vi "MCP4725 Generate and Read Example 4.vi"(8 "Error In":errorcluster) -> (0 "Error Out":errorcluster)   [LabVIEW 2014]
doc: "This example produces stepped triangle wave on output in loop, there's no timing inside while loop so it's running as fast as it can, at test computer signal has frequency 440Hz and consists from 12 samples, so we are able to produce this fast signals at most."
uses:
  LabVIEW-Universal-Transcriptor-MCP4725/MCP4725.lvclass
  <vilib>/LabVIEW Universal Transcriptor/LabVIEW to Arduino Transcriptor/Transcriptors/System API/Serial println string.vi
panel:
  # "This example produces stepped triangle wave on output in loop, there's no timing inside while loop so it's running as fast as it can, at test computer signal has frequency 440Hz and consists from 12 samples, so we are able to produce this fast signals at most.\n\nWiring:\n  Arduino Nano  |  MCP4725 module\n  -----------------------------------------\n          VCC        |           +5V\n          GND        |           GND\n          A4           |           SDA\n          A5           |           SCL"
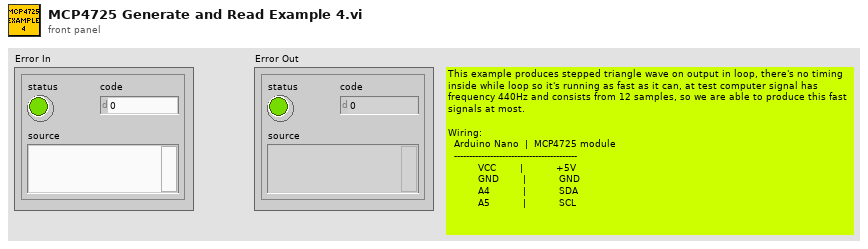
[diagram p1: front panel]
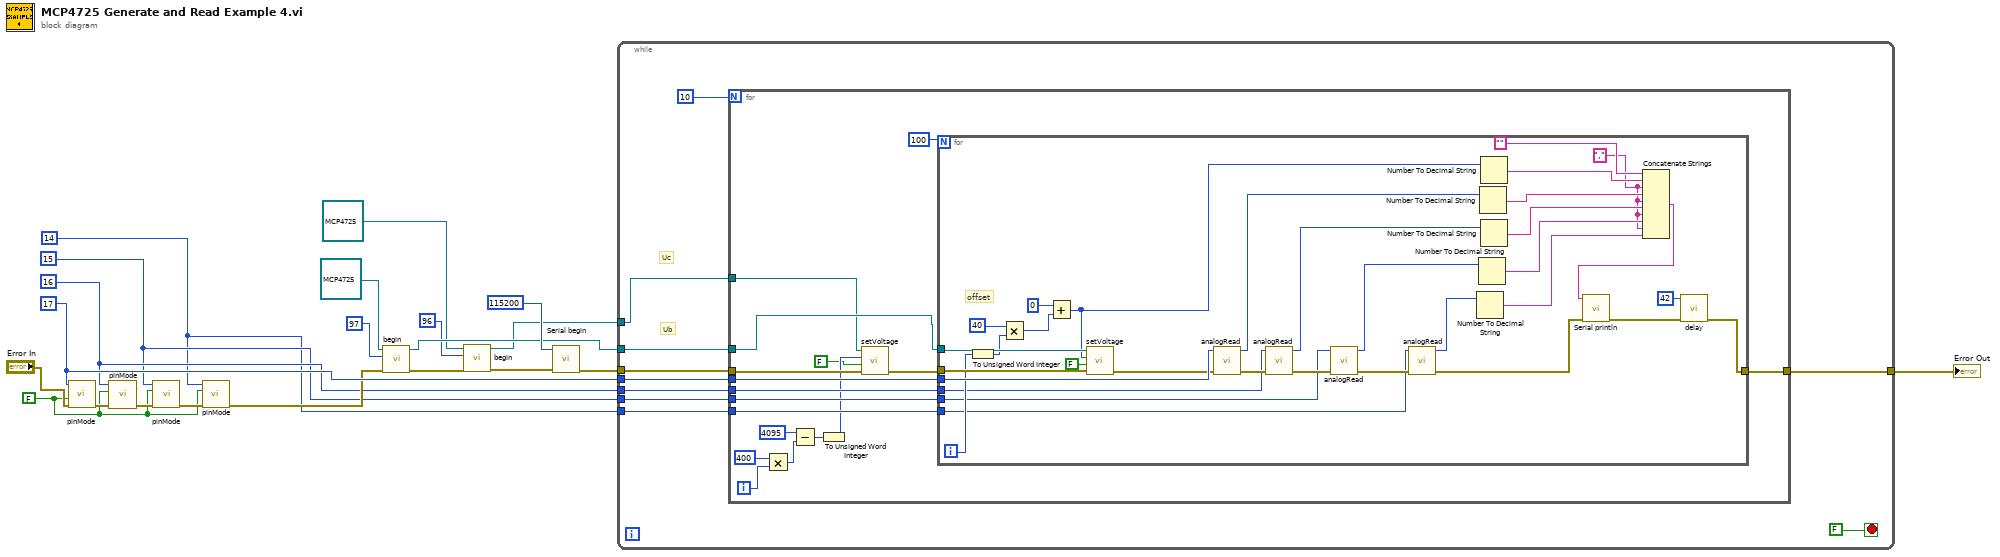
[diagram p0: block diagram]
diagram:
  w7 = 14 ("pin number")
  w8 = 15 ("pin number")
  w9 = 16 ("pin number")
  w11 = FALSE ("output?")
  w17 = 17 ("pin number")
  n1 = call <vilib>:"pinMode.vi"("Error In"="Error In", "output?"=w11, "pin number"=w17) -> ("Error Out"=w14:errorcluster)  [unwired: 8 in]
  n2 = call <vilib>:"pinMode.vi"("Error In"=w14, "output?"=w11, "pin number"=w9) -> ("Error Out"=w13:errorcluster)  [unwired: 8 in]
  n3 = call <vilib>:"pinMode.vi"("Error In"=w13, "output?"=w11, "pin number"=w8) -> ("Error Out"=w12:errorcluster)  [unwired: 8 in]
  n4 = call <vilib>:"pinMode.vi"("Error In"=w12, "output?"=w11, "pin number"=w7) -> ("Error Out"=w10:errorcluster)  [unwired: 8 in]
  n5 = call "begin.vi"("error in (no error)"=w10, "I2C addr"=u8 97, "MCP4725 in"=refnum<class "MCP4725.lvclass"> refnum) -> ("error out"=w6:errorcluster, "MCP4725 out"=w5:refnum<class "MCP4725.lvclass">)  [unwired: 7 in]
  n6 = call "begin.vi"("error in (no error)"=w6, "I2C addr"=u8 96, "MCP4725 in"=refnum<class "MCP4725.lvclass"> refnum) -> ("error out"=w2:errorcluster, "MCP4725 out"=w1:refnum<class "MCP4725.lvclass">)  [unwired: 7 in]
  n7 = call <vilib>:"Serial begin.vi"("Error In"=w2, "speed (Bd)"=115200) -> ("Error Out"=w16:errorcluster)  [unwired: 9 in]
  n8 = while {
    tunnel: w16 -> [w30]
    tunnel: w5 -> [w29]
    tunnel: [w28] -> w20
    tunnel: w17 -> [w27]
    tunnel: w9 -> [w26]
    tunnel: w8 -> [w25]
    tunnel: w7 -> [w24]
    tunnel: w1 -> [w23]
    stop <- FALSE stop-if-true
    # "Uc"
    # "Ub"
    n9 = for {
      N: 10 -> [_]
      tunnel: w29 -> [w33]
      tunnel: w27 -> [w47]
      tunnel: w26 -> [w45]
      tunnel: w25 -> [w44]
      tunnel: w24 -> [w43]
      tunnel: w23 -> [w32]
      tunnel: w30 -> [w42]
      tunnel: [w48] -> w28
      i -> [w38]
      n10 = Multiply(x=400, y=w38) -> (x*y=w39:i32)
      n11 = Subtract(x=4095, y=w39) -> (x-y=w36:i32)
      n12 = To Unsigned Word Integer(number=w36) -> (unsigned 16bit integer=w35:u16)
      n13 = call "setVoltage.vi"("error in (no error)"=w42, "writeEEPROM?"=FALSE, "voltage"=w35, "MCP4725 in"=w32) -> ("error out"=w41:errorcluster)  [unwired: 6 in, 1 out]
      n14 = for {
        N: 100 -> [_]
        tunnel: w41 -> [w81]
        tunnel: w33 -> [w80]
        tunnel: [w72] -> w48
        tunnel: w47 -> [w79]
        tunnel: w45 -> [w64]
        tunnel: w44 -> [w63]
        tunnel: w43 -> [w62]
        i -> [w74]
        w55 = "," ("string")
        # "offset"
        n15 = To Unsigned Word Integer(number=w74) -> (unsigned 16bit integer=w49:u16)
        n16 = Multiply(x=u16 40, y=w49) -> (x*y=w51:u16)
        n17 = Add(x=u16 0, y=w51) -> (x+y=w52:u16)
        n18 = call "setVoltage.vi"("error in (no error)"=w81, "writeEEPROM?"=FALSE, "voltage"=w52, "MCP4725 in"=w80) -> ("error out"=w54:errorcluster)  [unwired: 6 in, 1 out]
        n19 = call <vilib>:"analogRead.vi"("Error In"=w54, "pin number"=w79) -> ("Error Out"=w69:errorcluster, "value"=w68:u16)  [unwired: 8 in]
        n20 = call <vilib>:"analogRead.vi"("Error In"=w69, "pin number"=w64) -> ("Error Out"=w67:errorcluster, "value"=w61:u16)  [unwired: 8 in]
        n21 = call <vilib>:"analogRead.vi"("Error In"=w67, "pin number"=w63) -> ("Error Out"=w66:errorcluster, "value"=w60:u16)  [unwired: 8 in]
        n22 = call <vilib>:"analogRead.vi"("Error In"=w66, "pin number"=w62) -> ("Error Out"=w65:errorcluster, "value"=w59:u16)  [unwired: 8 in]
        n23 = Number To Decimal String(number=w59) -> (decimal integer string=w56:string)  [unwired: 1 in]
        n24 = Number To Decimal String(number=w60) -> (decimal integer string=w57:string)  [unwired: 1 in]
        n25 = Number To Decimal String(number=w68) -> (decimal integer string=w76:string)  [unwired: 1 in]
        n26 = Number To Decimal String(number=w52) -> (decimal integer string=w78:string)  [unwired: 1 in]
        n27 = Number To Decimal String(number=w61) -> (decimal integer string=w58:string)  [unwired: 1 in]
        n28 = Concatenate Strings("" ("string"), w78, w55, w76, w55, w58, w55, w57, w55, w56) -> (w75:string)
        n29 = call-poly <vilib>:"Serial println.vi"("Error In"=w65, "string in"=w75) -> ("Error Out"=w73:errorcluster)  [unwired: 9 in]
        n30 = call <vilib>:"delay.vi"("Error In"=w73, "time (ms)"=42) -> ("Error Out"=w72:errorcluster)  [unwired: 9 in]
      }
    }
  }
  "Error Out" <- w20
